vi "Heat1D_Solve Equations.vi"(5 "BC Type":i32, 7 "Coeff Array":dbl[](array[numeric]), 8 "Pivot":i32[](array[numeric]), 9 "U":T1, 10 "L":dbl[](array[numeric]), 11 "RHS":dbl[](array[numeric])) -> (3 "Solution Vector":dbl[](array[numeric]))   [LabVIEW 2020, in "NI_PDE.lvlib"]
uses:
  <vilib>/gmath/NI_PDE.lvlib
  <vilib>/Analysis/7linalg.llb/Solve Linear Equations (single right hand).vi
  <vilib>/Analysis/baseanly.llb/Solve Linear Equations By Cholesky.vi
  <vilib>/Analysis/baseanly.llb/Real Matrix to Compact Array.vi
  <vilib>/Analysis/baseanly.llb/Real Compact Tri-Matrix Linear Eqs.vi
  <vilib>/Analysis/7linalg.llb/Solve Linear Eqs (General).vi
  <vilib>/Analysis/7linalg.llb/Solve Linear Eqs (Gen, single right hand).vi
  <vilib>/Analysis/NI_AALPro.lvlib
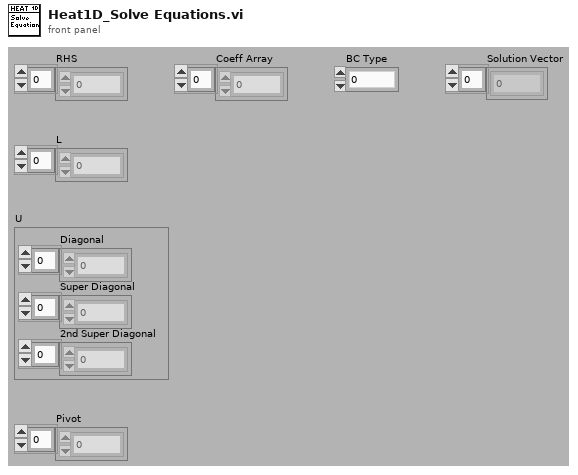
[diagram p1: front panel]
types:
  T1 = cluster{"Diagonal":dbl[], "Super Diagonal":dbl[], "2nd Super Diagonal":dbl[]}
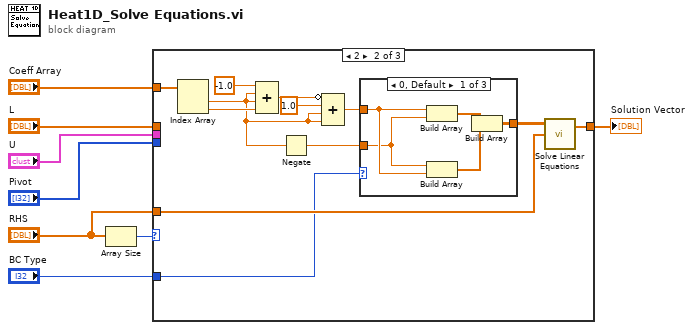
[diagram p0: block diagram]
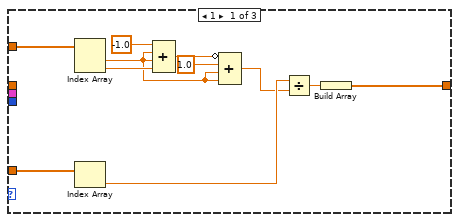
[diagram p2: hidden frame]
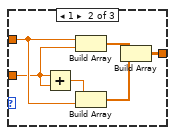
[diagram p3: hidden frame]
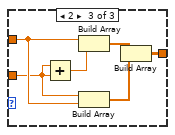
[diagram p4: hidden frame]
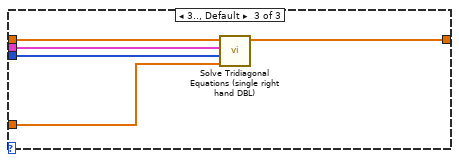
[diagram p5: hidden frame]
diagram:
  n1 = Array Size(array="RHS") -> (size(s)=w3:i32)
  n2 = case shown="2" w3 {
    tunnel: [w9 w21 w53] -> w8
    tunnel: "Pivot" -> [_ _ w52]
    tunnel: "U" -> [_ _ w51]
    tunnel: "L" -> [_ _ w50]
    tunnel: "RHS" -> [w19 w22 w49]
    tunnel: "Coeff Array" -> [w18 w31 _]
    tunnel: "BC Type" -> [_ w20 _]
    frame 1 {
      n3 = Index Array(array=w18) -> (element #1=w14:dbl, element #2=w17:dbl)  [unwired: 2 in]
      n4 = Index Array(array=w19) -> (element=w12:dbl)  [unwired: 1 in]
      n5 = Compound Arithmetic op=ADD(-1.0 ("value"), w14, w14, w17) -> (w15:dbl)
      n6 = Compound Arithmetic op=ADD(invert w15, 1.0 ("value"), w14, w14) -> (w11:dbl)
      n7 = Divide(x=w12, y=w11) -> (x/y=w10:dbl)
      n8 = Build Array(w10) -> (w9:dbl[])
    }
    frame 2 {
      n9 = Index Array(array=w31) -> (element #1=w26:dbl, element #2=w30:dbl)  [unwired: 2 in]
      n10 = Compound Arithmetic op=ADD(-1.0 ("value"), w26, w26, w30) -> (w28:dbl)
      n11 = Negate(x=w26) -> (-x=w25:dbl)
      n12 = Compound Arithmetic op=ADD(invert w28, 1.0 ("value"), w26, w26) -> (w24:dbl)
      n13 = case shown="0, Default" w20 {
        tunnel: w25 -> [w32 w38 w44]
        tunnel: w24 -> [w36 w42 w48]
        tunnel: [w33 w39 w45] -> w23
        frame 0, Default {
          n14 = Build Array(w36, w32) -> (w35:dbl[])
          n15 = Build Array(w32, w36) -> (w34:dbl[])
          n16 = Build Array(w35, w34) -> (w33:dbl[][])
        }
        frame 1 {
          n17 = Add(x=w38, y=w38) -> (x+y=w37:dbl)
          n18 = Build Array(w42, w38) -> (w41:dbl[])
          n19 = Build Array(w37, w42) -> (w40:dbl[])
          n20 = Build Array(w41, w40) -> (w39:dbl[][])
        }
        frame 2 {
          n21 = Add(x=w44, y=w44) -> (x+y=w43:dbl)
          n22 = Build Array(w48, w43) -> (w47:dbl[])
          n23 = Build Array(w44, w48) -> (w46:dbl[])
          n24 = Build Array(w47, w46) -> (w45:dbl[][])
        }
      }
      n25 = call-poly <vilib>:"Solve Linear Equations.vi"("Known Vector"=w22, "Input Matrix"=w23) -> ("Solution Vector"=w21:dbl[])  [unwired: 1 in, 1 out]
    }
    frame 3.., Default {
      n26 = call <vilib>:"Solve Tridiagonal Equations (single right hand DBL).vi"("Known Vector"=w49, "Pivot"=w52, "U"=w51, "L"=w50) -> ("Solution Vector"=w53:dbl[])  [unwired: 7 out]
    }
  }
  "Solution Vector" <- w8
